vi "Init.vi"(8 "error in (no error)":errorcluster, 11 "Simple Device in":refnum<class "Simple Device.lvclass">) -> (0 "error out":errorcluster, 3 "Simple Device out":refnum<class "Simple Device.lvclass">)   [LabVIEW 2021, in "Simple Device.lvclass"]
uses:
  Simple Device.lvclass
  Simple Device.lvclass/Simple Device.ctl
  TALOS/TALOS_PPL.lvlibp
  Libraries/Virtual Device Simulator/DeviceSim.lvlibp/DeviceReference/Simple  Virtual Device.lvclass
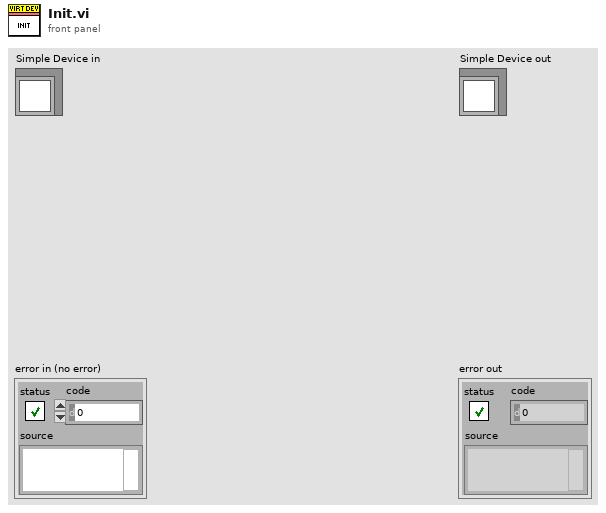
[diagram p1: front panel]
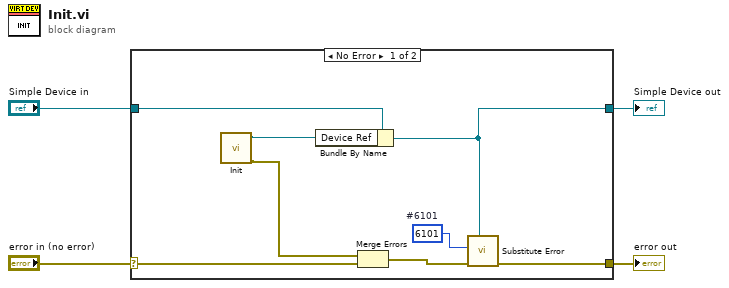
[diagram p0: block diagram]
diagram:
  n1 = case shown="No Error" "error in (no error)" {
    selector: "error in (no error)" -> [w10 w14]
    tunnel: [w8 w14] -> w3
    tunnel: [w11 w13] -> w1
    tunnel: "Simple Device in" -> [w12 w13]
    frame No Error {
      w7 = 6101  # #6101
      n2 = call "Init.vi"() -> ("error out"=w5:errorcluster, "Device Ref out"=w6:refnum<data-value>)  [unwired: 10 in]
      n3 = Bundle By Name(cluster=w12, "Device Ref"=w6) -> (w11:refnum<class "Simple Device.lvclass">)
      n4 = Merge Errors(w5, w10) -> (w9:errorcluster)
      n5 = call "Substitute Error.vi"("LabVIEW Object"=w11, "error in (no error)"=w9, "Error Code"=w7) -> ("error out"=w8:errorcluster)  [unwired: 8 in]
    }
    frame Error {
    }
  }
  "error out" <- w3
  "Simple Device out" <- w1
